vi "Start_Client_Coms.vi"(1 "VI name to run on server":string) -> (2 "LabVIEW application reference":refnum<vi>, 3 "Checked VI name":path, 4 "Local Call":bool, 5 "Error cluster":errorcluster)   [LabVIEW 2021]
uses:
  Anemometry/Anemometry Sub Vis/Controls/App_Global.ctl
  Anemometry/Anemometry Sub Vis/Controls/Server_Comms.ctl
  Anemometry/Anemometry Sub Vis/Globals/Dynamic_call_global.ph.vi
  Anemometry/Anemometry Sub Vis/Globals/Preference_global.vi
panel:
  out "Application:Exported VIs In Memory":string[](array[string])
  out "IP & Port No":string
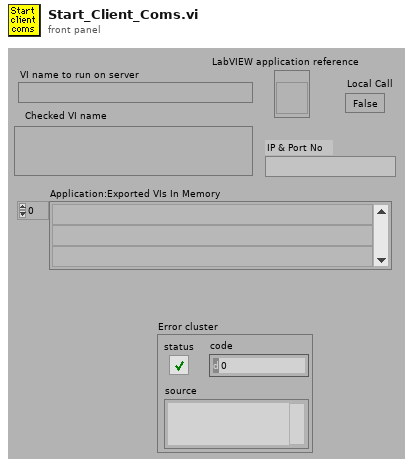
[diagram p1: front panel]
types:
  T1 = typedef "App_Global.ctl" = enum16{"Read Global", "Write to Global", "Initialise Array"}
  T2 = typedef "Server_Comms.ctl" = enum16{"Do Not Link To Server", "Server Link Healthy"}
  T3 = typedef "App_Ref_Cluster.ctl" = cluster{"Server IP & Port No":string, "Application reference":refnum<vi>}
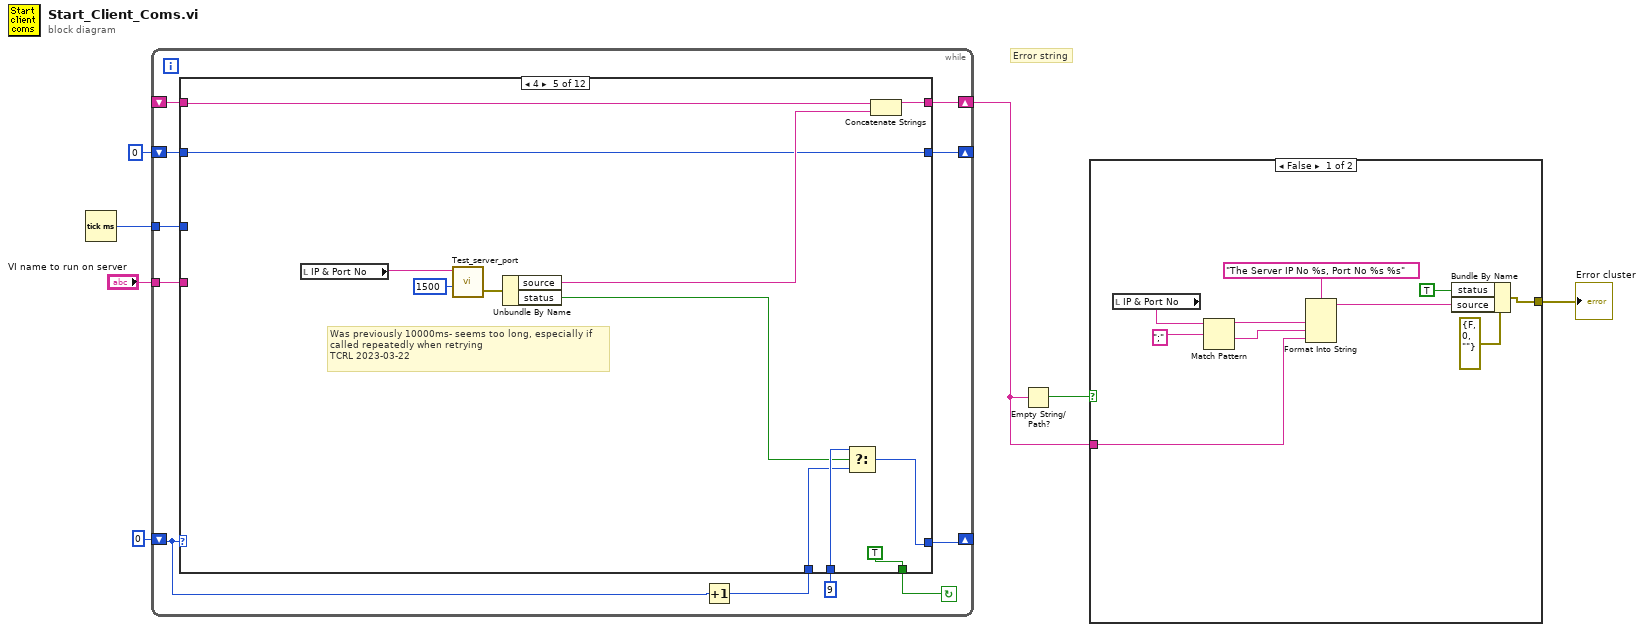
[diagram p0: block diagram]
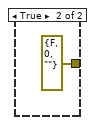
[diagram p2: hidden frame]
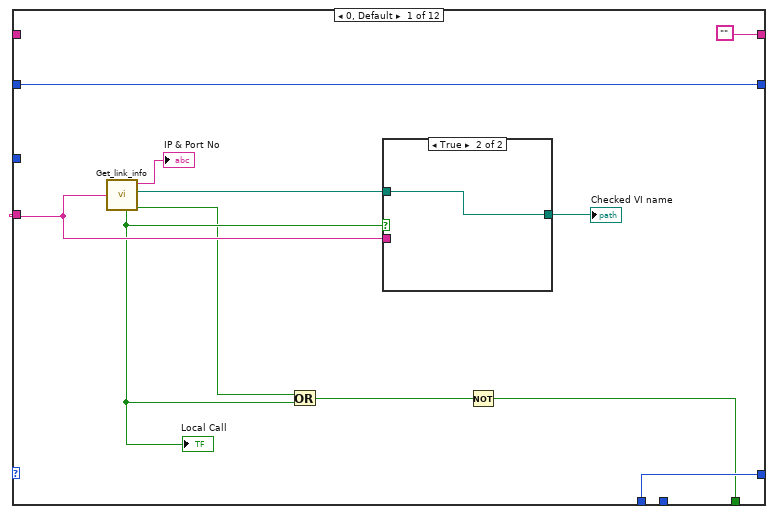
[diagram p3: hidden frame]
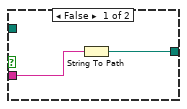
[diagram p4: hidden frame]
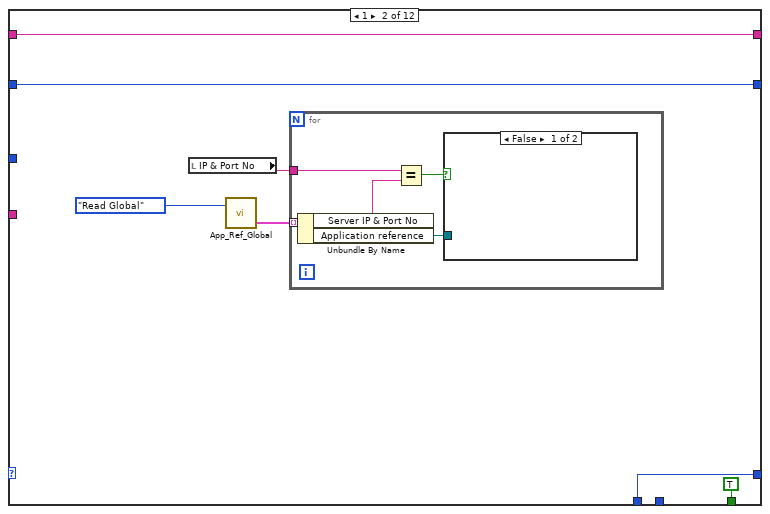
[diagram p5: hidden frame]
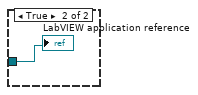
[diagram p6: hidden frame]
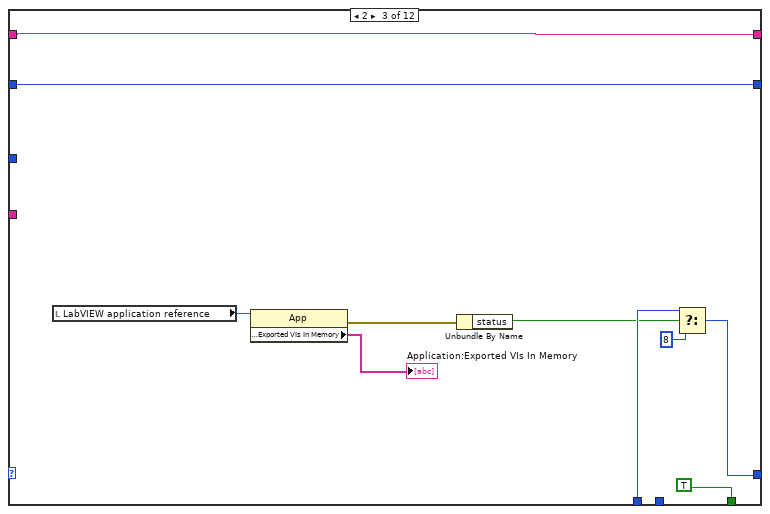
[diagram p7: hidden frame]
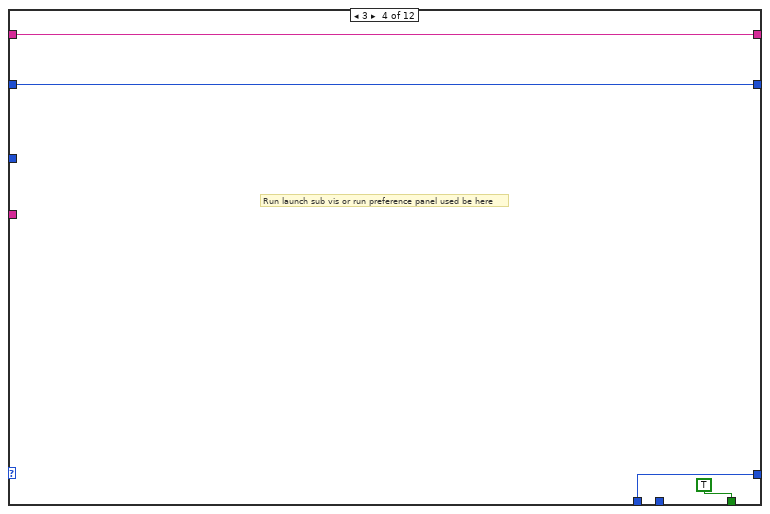
[diagram p8: hidden frame]
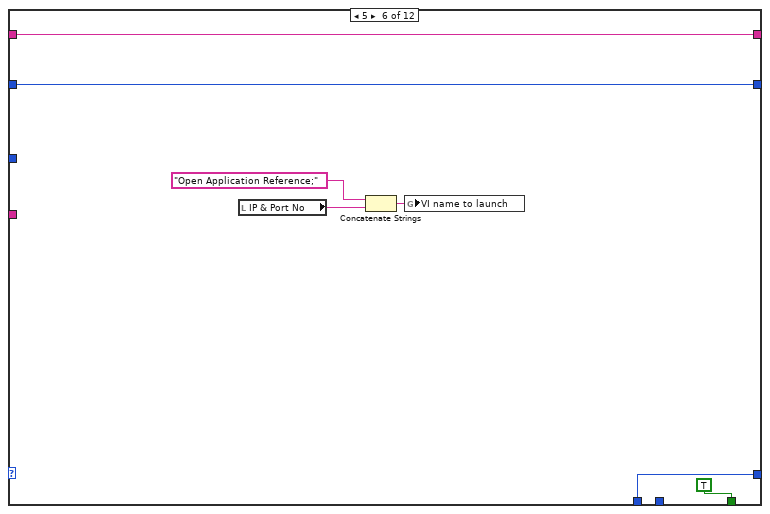
[diagram p9: hidden frame]
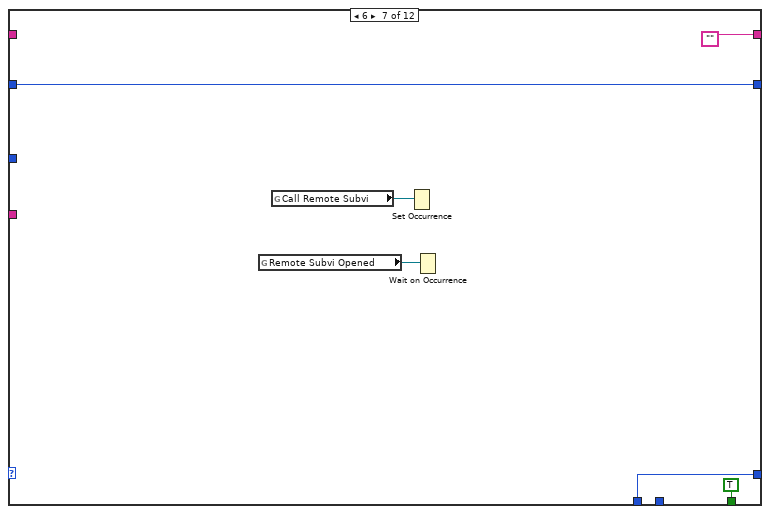
[diagram p10: hidden frame]
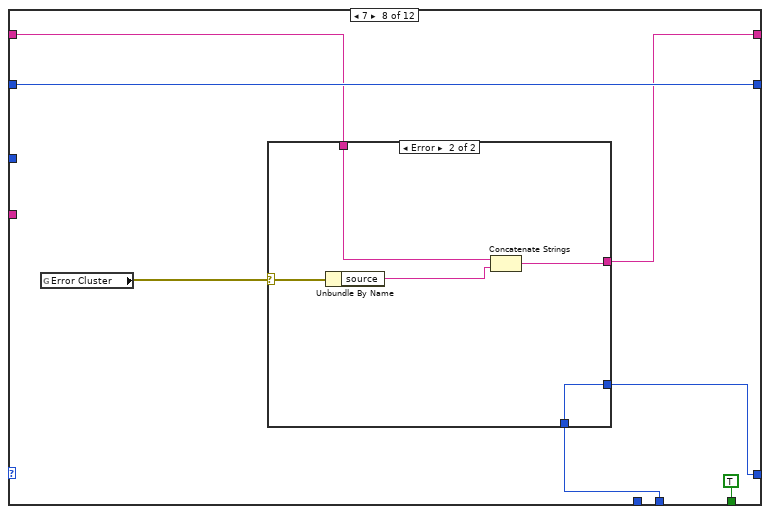
[diagram p11: hidden frame]
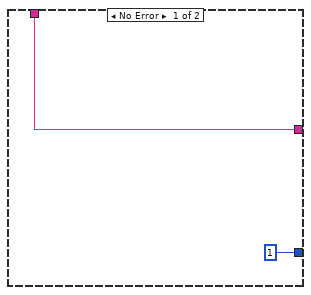
[diagram p12: hidden frame]
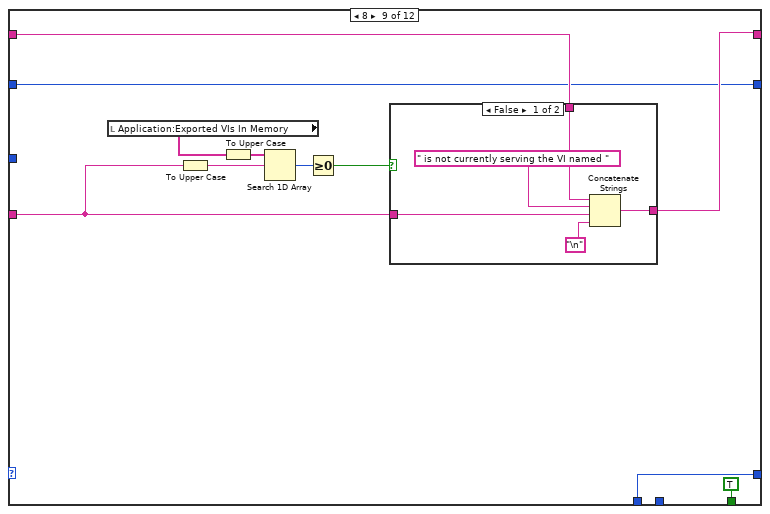
[diagram p13: hidden frame]
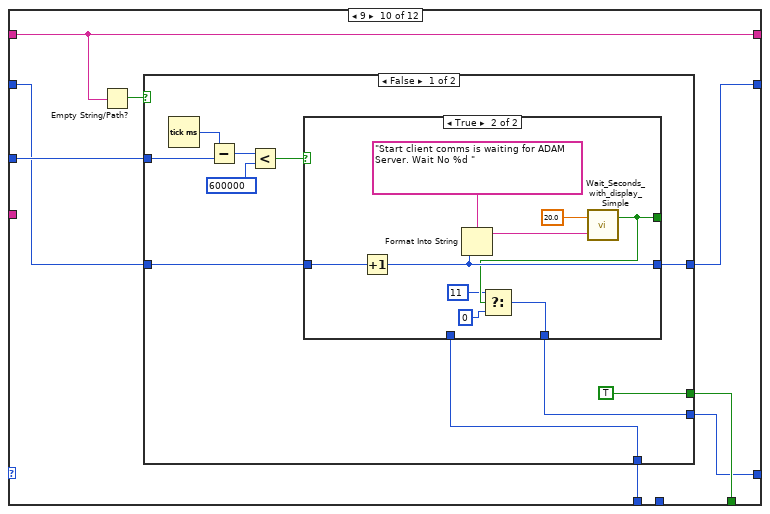
[diagram p15: hidden frame]
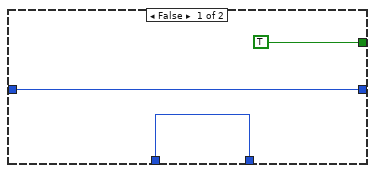
[diagram p16: hidden frame]
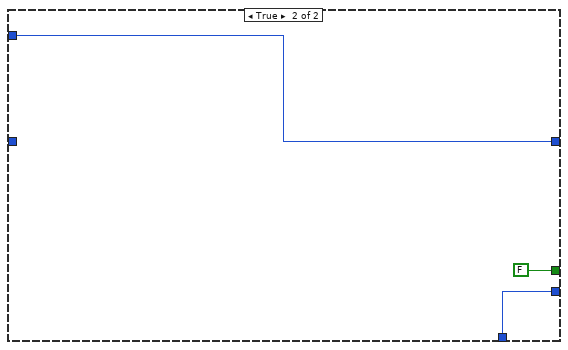
[diagram p17: hidden frame]
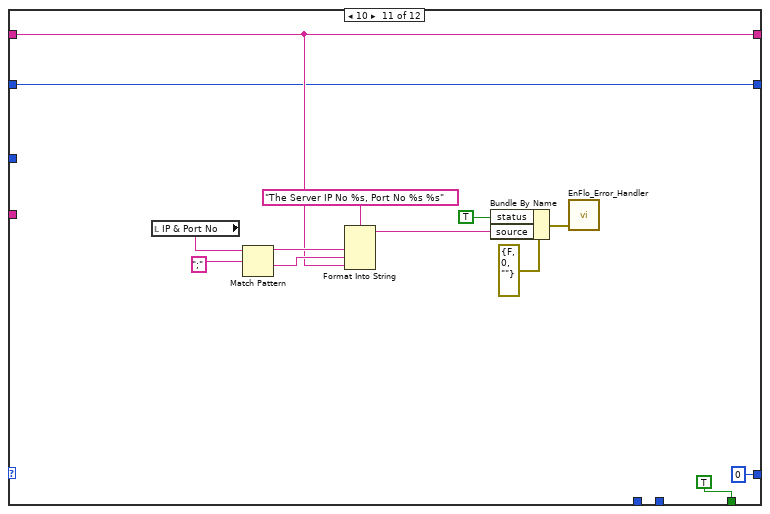
[diagram p18: hidden frame]
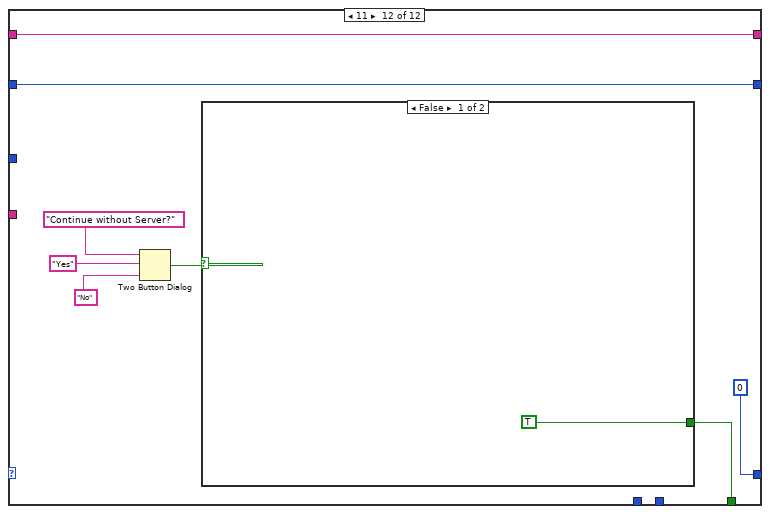
[diagram p19: hidden frame]
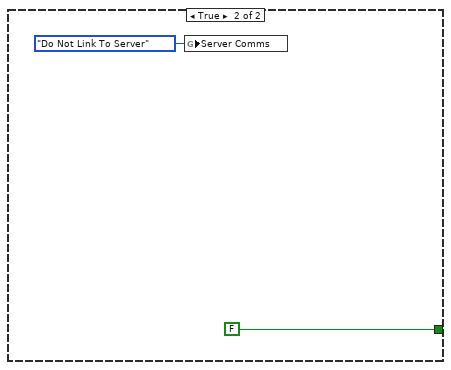
[diagram p20: hidden frame]
diagram:
  # "Error string"
  n1 = Tick Count (ms)() -> (millisecond timer value=w5:u32)
  n2 = while {
    shift-left: _ -> [w12]
    shift-right: [w13] -> w3
    shift-left: 0 -> [w16]
    shift-right: [w15] -> _
    tunnel: "VI name to run on server" -> [w17]
    tunnel: w5 -> [w10]
    shift-right: [w8] -> _
    shift-left: u32 0 ("millisecond timer value") -> [w9]
    stop <- w18 continue-if-true
    n3 = Increment(x=w16) -> (x+1=w14:i32)
    n4 = case shown="4" w16 {
      tunnel: [w24 TRUE ("status") TRUE ("status") TRUE ("status") TRUE ("status") TRUE ("status") TRUE ("status") TRUE ("status") TRUE ("status") w121 TRUE ("status") w163] -> w18
      tunnel: w17 -> [w26 _ _ _ _ _ _ _ w109 _ _ _]
      tunnel: [w28 w37 w52 w59 w65 w77 w80 w88 w102 w120 0 ("f") 0 ("f")] -> w15
      tunnel: w14 -> [w28 w37 w53 w59 w66 w77 w80 _ w102 w119 _ _]
      tunnel: ["" w35 w50 w57 w68 w76 "" w87 w100 w123 w153 w164] -> w13
      tunnel: w12 -> [_ w35 w50 w57 w69 w76 _ w86 w101 w123 w153 w164]
      tunnel: 9 ("f") -> [_ _ _ _ w67 _ _ w85 _ _ _ _]
      tunnel: w10 -> [_ _ _ _ _ _ _ _ _ w118 _ _]
      tunnel: w9 -> [w23 w33 w46 w56 w60 w72 w79 w90 w99 w117 w149 w169]
      tunnel: [w23 w33 w46 w56 w60 w72 w79 w90 w99 w116 w149 w169] -> w8
      frame 0, Default {
        n5 = call "Get_link_info.vi"("VI Name"=w26) -> ("badServer"=w19:bool, "Path name"=w25:path, "Server IP & Port"=→"IP & Port No":string, "Local Call?"=w21:bool)  [unwired: 1 out]
        "Local Call" <- w21
        n6 = Or(x=w19, y=w21) -> (x .or. y?=w20:bool)
        n7 = case shown="True" w21 {
          tunnel: [w30 w32] -> w29
          tunnel: w26 -> [w31 _]
          tunnel: w25 -> [_ w32]
          frame False {
            n8 = String To Path(string=w31) -> (path=w30:path)
          }
          frame True {
          }
        }
        "Checked VI name" <- w29
        n9 = Not(x=w20) -> (.not. x?=w24:bool)
      }
      frame 1 {
        n10 = local read "IP & Port No"() -> (w38:string)
        n11 = call "App_Ref_Global.vi"("Mode"=App_Global."Read Global") -> ("Output Array"=w39:T3[])  [unwired: 1 in, 1 out]
        n12 = for {
          tunnel: w39 -> [w44] mode=indexing
          tunnel: w38 -> [w42]
          n13 = Unbundle By Name(w44) -> ("Server IP & Port No"=w43:string, "Application reference"=w40:refnum<vi>)
          n14 = Equal?(x=w42, y=w43) -> (x = y?=w41:bool)
          n15 = case shown="False" w41 {
            tunnel: w40 -> [_ w45]
            frame False {
            }
            frame True {
              "LabVIEW application reference" <- w45
            }
          }
        }
      }
      frame 2 {
        n16 = local read "LabVIEW application reference"() -> (w55:refnum<vi>)
        n17 = property class="App"(reference=w55) -> (error out=w51:errorcluster, "Application:Exported VIs In Memory"=→"Application:Exported VIs In Memory":string[])  [unwired: 1 in, 1 out]
        n18 = Unbundle By Name(w51) -> ("status"=w48:bool)
        n19 = Select(t=w53, s=w48, f=8) -> (s? t:f=w52:i32)
      }
      frame 3 {
        # "Run launch sub vis or run preference panel used be here"
      }
      frame 4 {
        # "Was previously 10000ms- seems too long, especially if called repeatedly when retrying\nTCRL 2023-03-22"
        n20 = local read "IP & Port No"() -> (w62:string)
        n21 = call "Test_server_port.vi"("IP & Port No"=w62, "timeout ms (60000)"=1500) -> ("error out"=w61:errorcluster)  [unwired: 1 in, 3 out]
        n22 = Unbundle By Name(w61) -> ("source"=w70:string, "status"=w64:bool)
        n23 = Select(t=w67, s=w64, f=w66) -> (s? t:f=w65:i32)
        n24 = Concatenate Strings(w69, w70) -> (w68:string)
      }
      frame 5 {
        n25 = local read "IP & Port No"() -> (w74:string)
        n26 = Concatenate Strings("Open Application Reference;", w74) -> (w73:string)
        n27 = global write "Dynamic_call_global.ph.vi" "VI name to launch"(w73) -> ()
      }
      frame 6 {
        n28 = global read "Dynamic_call_global.ph.vi" "Remote Subvi Opened"() -> (w83:refnum<k4>)
        n29 = global read "Dynamic_call_global.ph.vi" "Call Remote Subvi"() -> (w82:refnum<k4>)
        n30 = Set Occurrence(w82) -> ()
        n31 = Wait on Occurrence(2:w83) -> ()  [unwired: 3 out]
      }
      frame 7 {
        n32 = global read "Dynamic_call_global.ph.vi" "Error Cluster"() -> (w89:errorcluster)
        n33 = case shown="Error" w89 {
          selector: w89 -> [_ w98]
          tunnel: [1 ("f") w94] -> w88
          tunnel: [w92 w96] -> w87
          tunnel: w86 -> [w92 w95]
          tunnel: w85 -> [_ w94]
          frame No Error {
          }
          frame Error {
            n34 = Unbundle By Name(w98) -> ("source"=w97:string)
            n35 = Concatenate Strings(w95, w97) -> (w96:string)
          }
        }
      }
      frame 8 {
        n36 = local read "Application:Exported VIs In Memory"() -> (w104:string[])
        n37 = To Upper Case(1:w109) -> (0:w108:string)
        n38 = To Upper Case(1:w104) -> (0:w107:string[])
        n39 = Search 1D Array(1D array=w107, element=w108) -> (index of element=w106:i32)  [unwired: 1 out]
        n40 = Greater Or Equal To 0?(x=w106) -> (x >= 0?=w105:bool)
        n41 = case shown="False" w105 {
          tunnel: w109 -> [w113 _]
          tunnel: w101 -> [w112 w115]
          tunnel: [w111 w115] -> w100
          frame False {
            n42 = Concatenate Strings(w112, " is not currently serving the VI named " ("Substring"), w113, "\n") -> (w111:string)
          }
          frame True {
          }
        }
      }
      frame 9 {
        n43 = Empty String/Path?(string/path=w123) -> (empty?=w122:bool)
        n44 = case shown="False" w122 {
          tunnel: [TRUE FALSE] -> w121
          tunnel: [w125 w147] -> w120
          tunnel: w119 -> [w124 w147]
          tunnel: w118 -> [w131 w146]
          tunnel: w117 -> [w127 _]
          tunnel: [w126 w146] -> w116
          frame False {
            n45 = Tick Count (ms)() -> (millisecond timer value=w132:u32)
            n46 = Subtract(x=w132, y=w131) -> (x-y=w130:u32)
            n47 = Less?(x=w130, y=u32 600000) -> (x < y?=w128:bool)
            n48 = case shown="True" w128 {
              tunnel: [TRUE ("Stopped") w140] -> _
              tunnel: w127 -> [w135 w143]
              tunnel: [w135 w141] -> w126
              tunnel: [w134 w138] -> w125
              tunnel: w124 -> [w134 _]
              frame False {
              }
              frame True {
                n49 = Increment(x=w143) -> (x+1=w141:u32)
                n50 = Format Into String(format string="Start client comms is waiting for ADAM Server. Wait No %d " ("Message"), w141) -> (resulting string=w142:string)  [unwired: 2 in, 1 out]
                n51 = call "Wait_Seconds_with_display_Simple.vi"("Message"=w142, "Seconds to wait"=20.0) -> ("Stopped"=w140:bool)  [unwired: 1 in]
                n52 = Select(t=11, s=w140, f=0 ("t")) -> (s? t:f=w138:i32)
              }
            }
          }
          frame True {
          }
        }
      }
      frame 10 {
        n53 = local read "IP & Port No"() -> (w161:string)
        n54 = Match Pattern(string=w161, regular expression=";") -> (before substring=w158:string, after substring=w157:string)  [unwired: 3 out]
        n55 = Format Into String(format string="The Server IP No %s, Port No %s %s" ("Format String"), w158, w157, w153) -> (resulting string=w152:string)  [unwired: 2 in, 1 out]
        n56 = Bundle By Name(cluster=errorcluster {"status"=FALSE, "code"=0, "source"=""} ("error in (no error)"), "status"=TRUE ("Bundle Element"), "source"=w152) -> (w154:errorcluster)
        n57 = call "EnFlo_Error_Handler.vi"("error in (no error)"=w154) -> ()  [unwired: 2 in, 3 out]
      }
      frame 11 {
        n58 = Two Button Dialog(message="Continue without Server?", 1:"No" ("F button name (\"Cancel\")"), 2:"Yes" ("T button name (\"OK\")")) -> (T button?=w165:bool)
        n59 = case shown="False" w165 {
          tunnel: [TRUE ("status") FALSE ("status")] -> w163
          frame False {
          }
          frame True {
            n60 = global write "Preference_global.vi" "Server Comms"(Server_Comms."Do Not Link To Server" ("Server Comms")) -> ()
          }
        }
      }
    }
  }
  n61 = Empty String/Path?(string/path=w3) -> (empty?=w1:bool)
  n62 = case shown="False" w1 {
    tunnel: w3 -> [w174 _]
    tunnel: [w173 errorcluster {"status"=FALSE, "code"=0, "source"=""} ("error in (no error)")] -> w2
    frame False {
      n63 = local read "IP & Port No"() -> (w175:string)
      n64 = Match Pattern(string=w175, regular expression=";") -> (before substring=w178:string, after substring=w179:string)  [unwired: 3 out]
      n65 = Format Into String(format string="The Server IP No %s, Port No %s %s" ("Format String"), w178, w179, w174) -> (resulting string=w182:string)  [unwired: 2 in, 1 out]
      n66 = Bundle By Name(cluster=errorcluster {"status"=FALSE, "code"=0, "source"=""} ("error in (no error)"), "status"=TRUE ("Bundle Element"), "source"=w182) -> (w173:errorcluster)
    }
    frame True {
    }
  }
  "Error cluster" <- w2
